vi "GlueSideDown.vi"() -> ()   [LabVIEW 2015]
uses:
  GlobalPath.vi
  GlobalData.vi
  GlobalVi.vi
panel:
  in  "ptfe 8":bool caption="Position the washer in the insert"
  in  "ptfe 7":bool caption="Deposit the glue with a thin needle on the emerging part of the alignment inserts/pins/slots"
  in  "ptfe 2":bool caption="Make sure the panel is rotated in such a way that the glued pins/inserts are facing downward"
  in  "ptfe 6":bool caption="Repeat the same procedure one more time to ensure that the glue is perfectly plane with respect to the PCB surface (solo sul O-ring)"
  out "PanelName":string
  in  "DONE ALL ?":bool
  in  "ptfe 5":bool caption="Wait 24h for the glue to cure"
  in  "ptfe 4":bool caption="Remove the excess glue using a small spatula"
  in  "ptfe 3":bool caption="Close the gap with Araldite 2011 glue using a thin syringe (coprire anche la parte di coverlay meta')"
  # "1. PCB gap closing side down"
  # "2. Washer gluing"
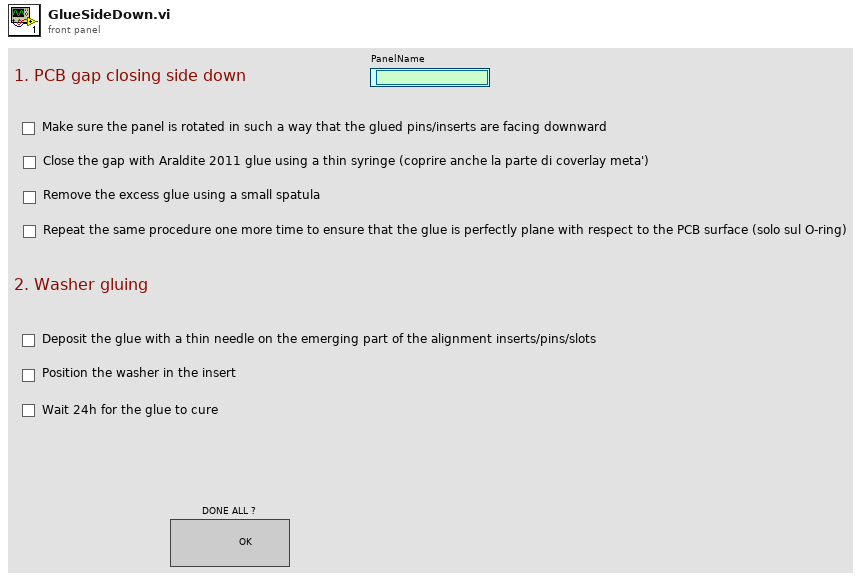
[diagram p1: front panel]
types:
  T1 = enum16{"open", "replace", "create", "open or create", "replace or create", "replace or create with confirmation"}
  T2 = enum32{"Bad", "Idle", "Run top level", "Running"}
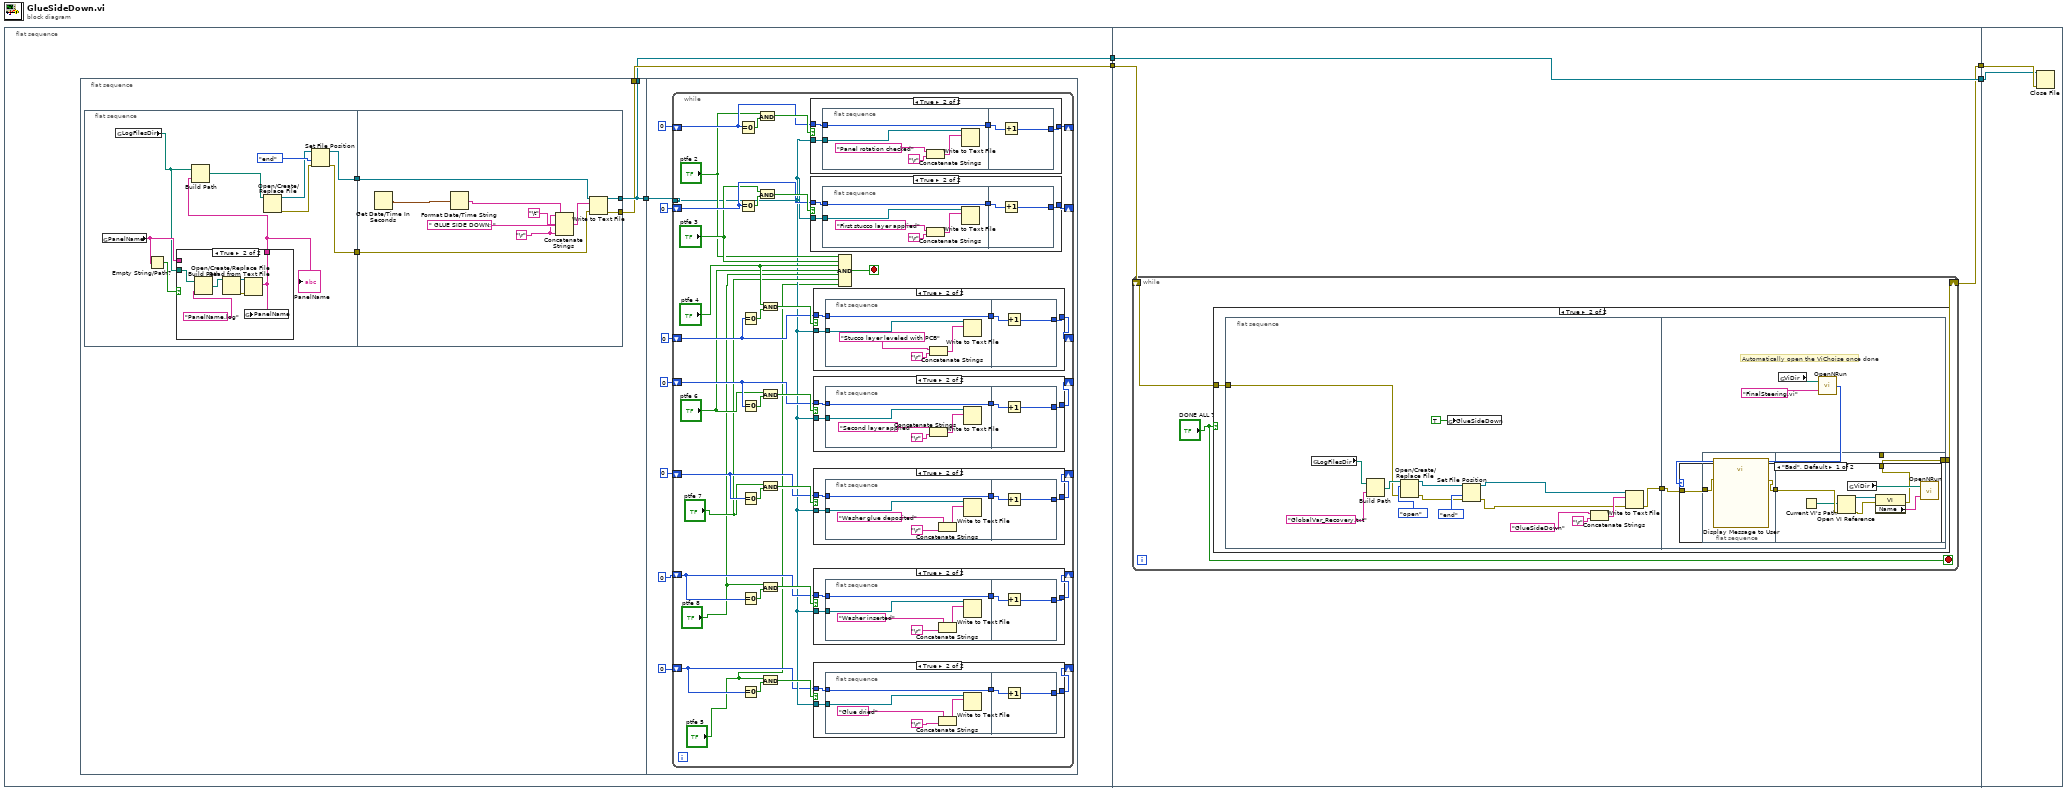
[diagram p0: block diagram]
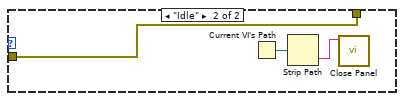
[diagram p11: hidden frame]
diagram:
  n1 = flat-sequence {
    tunnel: [w6] -> w3
    tunnel: [w5] -> w2
    tunnel: [w169] -> w4
    tunnel: w3 -> [w168]
    tunnel: w2 -> [w170]
    tunnel: [w170] -> w1
    tunnel: w4 -> [w214]
    tunnel: w1 -> [w213]
    frame #0 {
      n2 = flat-sequence {
        tunnel: [w10] -> w7
        tunnel: [w10] -> w5
        tunnel: [w9] -> w6
        tunnel: w7 -> [w46]
        frame #0 {
          n3 = flat-sequence {
            tunnel: [w16] -> w11
            tunnel: [w18] -> w8
            tunnel: w11 -> [w34]
            tunnel: [w33] -> w10
            tunnel: [w32] -> w9
            tunnel: w8 -> [w31]
            frame #0 {
              n4 = global read "GlobalData.vi" "PanelName"() -> (w15:string)
              n5 = global read "GlobalPath.vi" "LogFilesDir"() -> (w12:path)
              n6 = Empty String/Path?(string/path=w15) -> (empty?=w14:bool)
              n7 = case shown="True" w14 {
                tunnel: w12 -> [_ w28]
                tunnel: [w22 w23] -> w13
                tunnel: w15 -> [w22 _]
                frame False {
                }
                frame True {
                  n8 = Build Path(base path=w28, name or relative path="PanelName.log") -> (appended path=w27:path)
                  n9 = Open/Create/Replace File(file path (use dialog)=w27) -> (refnum out=w24:refnum<file>, error out=w25:errorcluster)  [unwired: 5 in, 1 out]
                  n10 = Read from Text File(file (use dialog)=w24, error in=w25) -> (text=w23:string)  [unwired: 2 in, 3 out]
                  n11 = global write "GlobalData.vi" "PanelName"(w23) -> ()
                }
              }
              "PanelName" <- w13
              n12 = Build Path(base path=w12, name or relative path=w13) -> (appended path=w21:path)
              n13 = Open/Create/Replace File(file path (use dialog)=w21) -> (refnum out=w17:refnum<file>, error out=w19:errorcluster)  [unwired: 5 in, 1 out]
              n14 = Set File Position(refnum=w17, from (0:start)=enum16{"start", "end", "current"}."end", error in=w19) -> (refnum out=w16:refnum<file>, error out=w18:errorcluster)  [unwired: 1 in]
            }
            frame #1 {
              w29 = "\r"
              n15 = Get Date/Time In Seconds() -> (seconds since 1Jan1904=w30:timestamp)
              n16 = Format Date/Time String(seconds (now)=w30) -> (date/time string=w36:string)  [unwired: 2 in]
              n17 = Concatenate Strings(w29, w36, "\t", " GLUE SIDE DOWN: ", w29) -> (w35:string)
              n18 = Write to Text File(file (use dialog)=w34, text=w35, error in=w31) -> (refnum out=w33:refnum<file>, error out=w32:errorcluster)  [unwired: 1 in, 1 out]
            }
          }
        }
        frame #1 {
          n19 = while {
            tunnel: w46 -> [w50]
            shift-right: [w79] -> _
            shift-left: 0 -> [w80]
            shift-right: [w75] -> _
            shift-left: 0 -> [w76]
            shift-right: [w69] -> _
            shift-left: 0 -> [w71]
            shift-right: [w65] -> _
            shift-left: 0 -> [w66]
            shift-right: [w61] -> _
            shift-left: 0 -> [w62]
            shift-right: [w57] -> _
            shift-left: 0 -> [w58]
            shift-right: [w48] -> _
            shift-left: 0 -> [w49]
            stop <- w83 stop-if-true
            n20 = Equal To 0?(x=w80) -> (x = 0?=w82:bool)
            n21 = Equal To 0?(x=w76) -> (x = 0?=w78:bool)
            n22 = Equal To 0?(x=w71) -> (x = 0?=w73:bool)
            n23 = Equal To 0?(x=w66) -> (x = 0?=w68:bool)
            n24 = Equal To 0?(x=w58) -> (x = 0?=w60:bool)
            n25 = Equal To 0?(x=w62) -> (x = 0?=w64:bool)
            n26 = Equal To 0?(x=w49) -> (x = 0?=w52:bool)
            n27 = And(x="ptfe 2", y=w82) -> (x .and. y?=w81:bool)
            n28 = And(x="ptfe 3", y=w78) -> (x .and. y?=w77:bool)
            n29 = And(x="ptfe 4", y=w73) -> (x .and. y?=w72:bool)
            n30 = And(x="ptfe 6", y=w68) -> (x .and. y?=w67:bool)
            n31 = And(x="ptfe 7", y=w60) -> (x .and. y?=w59:bool)
            n32 = And(x="ptfe 8", y=w64) -> (x .and. y?=w63:bool)
            n33 = And(x="ptfe 5", y=w52) -> (x .and. y?=w51:bool)
            n34 = case shown="True" w81 {
              tunnel: w50 -> [_ w160]
              tunnel: w80 -> [w156 w158]
              tunnel: [w156 w157] -> w79
              frame False {
              }
              frame True {
                n35 = flat-sequence {
                  tunnel: w160 -> [w163]
                  tunnel: [w162] -> w159
                  tunnel: w158 -> [w162]
                  tunnel: w159 -> [w167]
                  tunnel: [w166] -> w157
                  frame #0 {
                    n36 = Concatenate Strings("Panel rotation checked", "\r") -> (w165:string)
                    n37 = Write to Text File(file (use dialog)=w163, text=w165) -> ()  [unwired: 2 in, 3 out]
                  }
                  frame #1 {
                    n38 = Increment(x=w167) -> (x+1=w166:i32)
                  }
                }
              }
            }
            n39 = case shown="True" w77 {
              tunnel: w50 -> [_ w148]
              tunnel: w76 -> [w144 w146]
              tunnel: [w144 w145] -> w75
              frame False {
              }
              frame True {
                n40 = flat-sequence {
                  tunnel: w148 -> [w151]
                  tunnel: [w150] -> w147
                  tunnel: w146 -> [w150]
                  tunnel: w147 -> [w155]
                  tunnel: [w154] -> w145
                  frame #0 {
                    n41 = Concatenate Strings("First stucco layer applied", "\r") -> (w153:string)
                    n42 = Write to Text File(file (use dialog)=w151, text=w153) -> ()  [unwired: 2 in, 3 out]
                  }
                  frame #1 {
                    n43 = Increment(x=w155) -> (x+1=w154:i32)
                  }
                }
              }
            }
            n44 = case shown="True" w72 {
              tunnel: w50 -> [_ w136]
              tunnel: w71 -> [w132 w134]
              tunnel: [w132 w133] -> w69
              frame False {
              }
              frame True {
                n45 = flat-sequence {
                  tunnel: w136 -> [w139]
                  tunnel: [w138] -> w135
                  tunnel: w134 -> [w138]
                  tunnel: w135 -> [w143]
                  tunnel: [w142] -> w133
                  frame #0 {
                    n46 = Concatenate Strings("Stucco layer leveled with PCB", "\r") -> (w141:string)
                    n47 = Write to Text File(file (use dialog)=w139, text=w141) -> ()  [unwired: 2 in, 3 out]
                  }
                  frame #1 {
                    n48 = Increment(x=w143) -> (x+1=w142:i32)
                  }
                }
              }
            }
            n49 = case shown="True" w67 {
              tunnel: w50 -> [_ w124]
              tunnel: w66 -> [w120 w122]
              tunnel: [w120 w121] -> w65
              frame False {
              }
              frame True {
                n50 = flat-sequence {
                  tunnel: w124 -> [w127]
                  tunnel: [w126] -> w123
                  tunnel: w122 -> [w126]
                  tunnel: w123 -> [w131]
                  tunnel: [w130] -> w121
                  frame #0 {
                    n51 = Concatenate Strings("Second layer applied", "\r") -> (w129:string)
                    n52 = Write to Text File(file (use dialog)=w127, text=w129) -> ()  [unwired: 2 in, 3 out]
                  }
                  frame #1 {
                    n53 = Increment(x=w131) -> (x+1=w130:i32)
                  }
                }
              }
            }
            n54 = case shown="True" w59 {
              tunnel: w50 -> [_ w100]
              tunnel: w58 -> [w96 w98]
              tunnel: [w96 w97] -> w57
              frame False {
              }
              frame True {
                n55 = flat-sequence {
                  tunnel: w100 -> [w103]
                  tunnel: [w102] -> w99
                  tunnel: w98 -> [w102]
                  tunnel: w99 -> [w107]
                  tunnel: [w106] -> w97
                  frame #0 {
                    n56 = Concatenate Strings("Washer glue deposited", "\r") -> (w105:string)
                    n57 = Write to Text File(file (use dialog)=w103, text=w105) -> ()  [unwired: 2 in, 3 out]
                  }
                  frame #1 {
                    n58 = Increment(x=w107) -> (x+1=w106:i32)
                  }
                }
              }
            }
            n59 = case shown="True" w63 {
              tunnel: w50 -> [_ w112]
              tunnel: w62 -> [w108 w110]
              tunnel: [w108 w109] -> w61
              frame False {
              }
              frame True {
                n60 = flat-sequence {
                  tunnel: w112 -> [w115]
                  tunnel: [w114] -> w111
                  tunnel: w110 -> [w114]
                  tunnel: w111 -> [w119]
                  tunnel: [w118] -> w109
                  frame #0 {
                    n61 = Concatenate Strings("Washer inserted", "\r") -> (w117:string)
                    n62 = Write to Text File(file (use dialog)=w115, text=w117) -> ()  [unwired: 2 in, 3 out]
                  }
                  frame #1 {
                    n63 = Increment(x=w119) -> (x+1=w118:i32)
                  }
                }
              }
            }
            n64 = case shown="True" w51 {
              tunnel: w50 -> [_ w88]
              tunnel: w49 -> [w84 w86]
              tunnel: [w84 w85] -> w48
              frame False {
              }
              frame True {
                n65 = flat-sequence {
                  tunnel: w88 -> [w91]
                  tunnel: [w90] -> w87
                  tunnel: w86 -> [w90]
                  tunnel: w87 -> [w95]
                  tunnel: [w94] -> w85
                  frame #0 {
                    n66 = Concatenate Strings("Glue dried", "\r") -> (w93:string)
                    n67 = Write to Text File(file (use dialog)=w91, text=w93) -> ()  [unwired: 2 in, 3 out]
                  }
                  frame #1 {
                    n68 = Increment(x=w95) -> (x+1=w94:i32)
                  }
                }
              }
            }
            n69 = Compound Arithmetic op=AND("ptfe 2", "ptfe 3", "ptfe 4", "ptfe 6", "ptfe 8", "ptfe 7", "ptfe 5") -> (w83:bool)
          }
        }
      }
    }
    frame #1 {
      n70 = while {
        shift-right: [w173] -> w169
        shift-left: w168 -> [w172]
        stop <- "DONE ALL ?" stop-if-true
        n71 = case shown="True" "DONE ALL ?" {
          tunnel: [w174 w177] -> w173
          tunnel: w172 -> [w174 w176]
          frame False {
          }
          frame True {
            n72 = flat-sequence {
              tunnel: w176 -> [w181]
              tunnel: [w180] -> w175
              tunnel: [w194] -> w177
              tunnel: w175 -> [w193]
              frame #0 {
                n73 = global read "GlobalPath.vi" "LogFilesDir"() -> (w178:path)
                n74 = Build Path(base path=w178, name or relative path="GlobalVar_Recovery.txt") -> (appended path=w190:path)
                n75 = Open/Create/Replace File(file path (use dialog)=w190, error in=w181, operation (0:open)=T1."open") -> (refnum out=w186:refnum<file>, error out=w187:errorcluster)  [unwired: 3 in, 1 out]
                n76 = global write "GlobalVi.vi" "GlueSideDown"(TRUE) -> ()
                n77 = Set File Position(refnum=w186, from (0:start)=enum16{"start", "end", "current"}."end", error in=w187) -> (refnum out=w183:refnum<file>, error out=w182:errorcluster)  [unwired: 1 in]
                n78 = Concatenate Strings("GlueSideDown", "\r") -> (w185:string)
                n79 = Write to Text File(file (use dialog)=w183, text=w185, error in=w182) -> (error out=w180:errorcluster)  [unwired: 1 in, 2 out]
              }
              frame #1 {
                # "Automatically open the ViChoise once done"
                n80 = global read "GlobalPath.vi" "ViDir"() -> (w197:path)
                n81 = call "OpenNRun.vi"("VI name"="FinalSteering.vi", "ViDirPath"=w197) -> ("Execution:State"=w196:T2)
                n82 = case shown="\"Bad\", Default" w196 {
                  tunnel: [w198 w210] -> w194
                  tunnel: w193 -> [w199 w210]
                  frame "Bad", Default {
                    n83 = flat-sequence {
                      tunnel: w199 -> [w202]
                      tunnel: [w201] -> w200
                      tunnel: w200 -> [w206]
                      tunnel: [w203] -> w198
                      frame #0 {
                        n84 = call "Display Message to User"("error in (no error)"=w202) -> ("error out"=w201:errorcluster)  [unwired: 9 in, 1 out]
                      }
                      frame #1 {
                        n85 = Current VI's Path() -> (path=w204:path)
                        n86 = Open VI Reference(vi path=w204, error in (no error)=w206) -> (vi reference=w209:refnum<vi>, error out=w208:errorcluster)  [unwired: 4 in]
                        n87 = global read "GlobalPath.vi" "ViDir"() -> (w205:path)
                        n88 = property class="VI"(reference=w209, error in=w208) -> (error out=w203:errorcluster, "Name"=w207:string)  [unwired: 1 out]
                        n89 = call "OpenNRun.vi"("VI name"=w207, "ViDirPath"=w205) -> ()  [unwired: 1 out]
                      }
                    }
                  }
                  frame "Idle" {
                    n90 = Current VI's Path() -> (path=w211:path)
                    n91 = Strip Path(path=w211) -> (name=w212:string)  [unwired: 1 out]
                    n92 = call <vilib>:"Close Panel.vi"("VI name"=w212) -> ()  [unwired: 10 in, 1 out]
                  }
                }
              }
            }
          }
        }
      }
    }
    frame #2 {
      n93 = Close File(refnum=w213, error in=w214) -> ()  [unwired: 2 out]
    }
  }
